vi "temperature_calc.vi"(9 "Sensor parameters":T1, 10 "proud":dbl, 11 "napeti":dbl) -> (0 "Odpor":dbl, 3 "teplota":dbl)   [LabVIEW 2021]
uses:
  controls/Sensor parameters.ctl
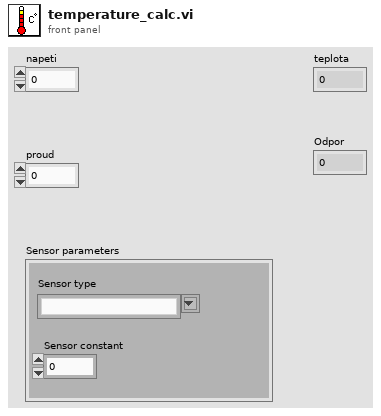
[diagram p1: front panel]
types:
  T1 = typedef "Sensor parameters.ctl" = cluster{"Sensor type":string, "Sensor constant":dbl}
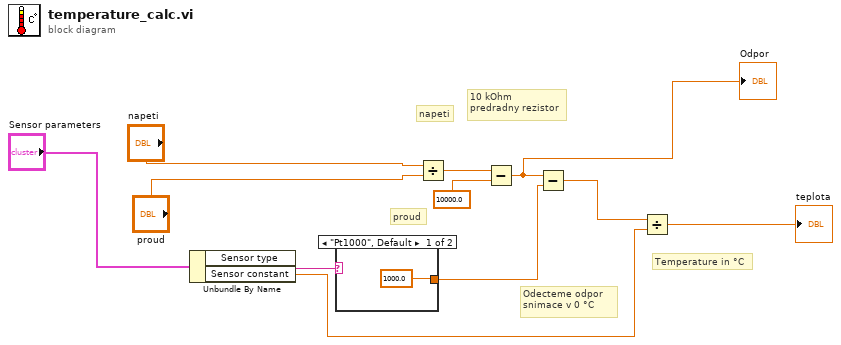
[diagram p0: block diagram]
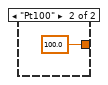
[diagram p2: hidden frame]
diagram:
  # "Temperature in °C"
  # "Odecteme odpor \nsnimace v 0 °C"
  # "10 kOhm \npredradny rezistor"
  # "proud"
  # "napeti"
  n1 = Unbundle By Name("Sensor parameters") -> ("Sensor type"=w7:string, "Sensor constant"=w10:dbl)
  n2 = case shown="\"Pt1000\", Default" w7 {
    tunnel: [1000.0 100.0] -> w8
    frame "Pt1000", Default {
    }
    frame "Pt100" {
    }
  }
  n3 = Divide(x="napeti", y="proud") -> (x/y=w4:dbl)
  n4 = Subtract(x=w4, y=10000.0) -> (x-y=w1:dbl)
  "Odpor" <- w1
  n5 = Subtract(x=w1, y=w8) -> (x-y=w9:dbl)
  n6 = Divide(x=w9, y=w10) -> (x/y=→"teplota":dbl)
